vi "PH_PILS.ProcCases.vi"(0 "i ref in":refnum<vi>, 1 "selector":string, 2 "Data":T1, 3 "call cluster":T2={"Object"="", "Selector"="", "CallType"=enum."synchronous", "Async Object"="", "Async Selector"="", "Data Descriptor"="", "Data"=[], "Error #"=0, "Expire"=0}, 5 "error in (no error)":errorcluster) -> (14 "i ref out":refnum<vi>, 17 "answer cluster":T2={"Object"="", "Selector"="", "CallType"=enum."synchronous", "Async Object"="", "Async Selector"="", "Data Descriptor"="", "Data"=[], "Error #"=0, "Expire"=0}, 19 "error out":errorcluster)   [LabVIEW 2014, in "PH_PILS.lvlib"]
doc: "This method is called by a process from within the default case in the event loop. The methods of a class that are linked to events will be called from THIS method. Add your code here."
uses:
  PH_PILS.lvlib
  CSCore/CSSystem/CoreDefs/CoreDefs.call_type.ctl
  CSCore/BaseProcess/BaseProcess.descriptor string definition.ctl
  CSCore/CSSystem/CoreDefs/CoreDefs.rawDataType.ctl
  PH_SystemInformation/PH_SystemInformationEnabling State.ctl
  PH_Beckhoff_PP_Control/PH_Beckhoff_PP_Control.PP Mercury Tags.ctl
  CSCore/CSSystem/CoreLib/CoreLib.string 2 byte array.vi
  CSCore/BaseProcess/BaseProcess.lvlib
  CSCore/CSSystem/CoreLib/CoreLib.lvlib
  CSCore/CAEObj/CAEObj.lvlib
  PH_Common/PH_Common.lvlib
  PH_SystemInformation/PH_SystemInformation.lvlib
  PH_StatusHandler/PH_StatusHandler.lvlib
  PH_Beckhoff_PP_Control/PH_Beckhoff_PP_Control.lvlib
  PH_Beckhoff/PH_Beckhoff.lvlib
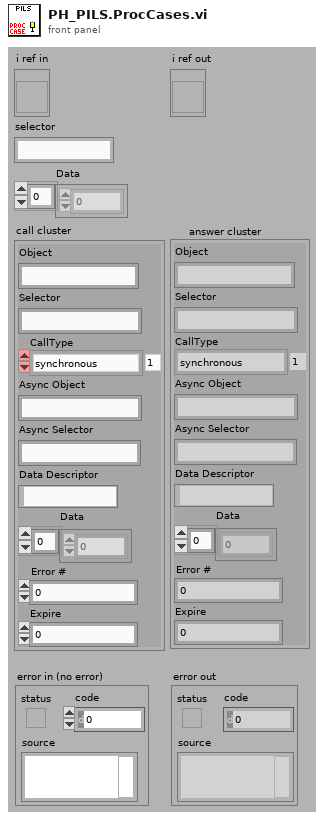
[diagram p1: front panel]
types:
  T1 = typedef "CoreDefs.rawDataType.ctl" = i8[]
  T2 = typedef "CoreDefs.call_type.ctl" = cluster{"Object":string, "Selector":string, "CallType":enum16{"simple", "synchronous", "asynchronous"}, "Async Object":string, "Async Selector":string, "Data Descriptor":T3, "Data":T1, "Error #":i32, "Expire":u32}
  T3 = typedef "BaseProcess.lvlib/BaseProcess.descriptor string definition.ctl" = string
  T4 = enum16{"unknown", "intern", "4 (Z6)", "3", "2", "1"}
  T5 = typedef "PH_Beckhoff_PP_Control.lvlib/PH_Beckhoff_PP_Control.PP Mercury Tags.ctl" = enum16{"Device-on", "Alarm", "on-since", "Concentration", "Status"}
  T6 = enum16{"Laser", "PreAmp", "MainAmp", "Exp 1", "Exp 2", "Exp 3", "Exp 4"}[]
  T7 = typedef "PH_SystemInformation.lvlib/PH_SystemInformationEnabling State.ctl" = i32
  T8 = typedef "PH_PILS.lvlib/PH_PILS.i attribute.ctl" = cluster{"Boolean":cluster{"GUI Ref":refnum<vi>, "Status":i32}[], "GUI Refs Exp. Shutters":cluster{"1":refnum<vi>, "2":refnum<vi>, "3":refnum<vi>, "4":refnum<vi>}, "Tristate2Run GUI Refs":refnum<vi>[], "EO-Likes":cluster{"GUI Ref":refnum<vi>, "Status":i32}[], "Operation Mode":cluster{"Operation Mode":T9, "GUI":cluster{"Ref State":refnum<vi>, "Ref":refnum<vi>}, "Servicemode":cluster{"Tagname":string, "Status":i32}, "Labormode":cluster{"Tagname":string, "Status":i32}, "Searchmode":cluster{"Tagname":string, "Status":i32}, "Shotmode":cluster{"Tagname":string, "Status":i32}}, "Submode":cluster{"Submode":T10, "GUI":cluster{"Ref State":refnum<vi>, "Ref":refnum<vi>}, "Submode":cluster{"Tagname":string, "Status":i32}}, "Experiment":cluster{"Experiment":enum16{"unknown", "intern", "4 (Z6)", "3", "2", "1"}, "GUI":cluster{"Ref State":refnum<vi>, "Ref":refnum<vi>}, "intern":cluster{"Tagname":string, "Status":i32}, "Exp 4":cluster{"Tagname":string, "Status":i32}, "Exp 3":cluster{"Tagname":string, "Status":i32}, "Exp 2":cluster{"Tagname":string, "Status":i32}, "Exp 1":cluster{"Tagname":string, "Status":i32}}, "TristateNormal":cluster{"GUI Ref":refnum<vi>, "Status":i32}[], "Door Tags":cluster{"GUI Ref":refnum<vi>, "Status":i32}[], "GUIlessTags":cluster{"Name":string, "Status":i32}[], "Beamline GUI Refs":refnum<vi>[], "Special Boolean":cluster{"GUI Ref":refnum<vi>, "Status":i32}[], "Laserpower":cluster{"GUI Ref":refnum<vi>, "Status":i32}[], "Shutter":cluster{"GUI Ref":refnum<vi>, "Status":i32}[], "Tristate EO Like":cluster{"GUI Ref":refnum<vi>, "Status":i32}[], "PP":cluster{"GUI Ref":refnum<vi>, "Status":i32, "Head Ref":refnum<vi>, "Slider Ref":refnum<vi>}[], "Switch Knobs":cluster{"GUI Ref":refnum<vi>, "Status":i32}[], "Latch Knob GUI Refs":refnum<vi>[], "FailureCounter":i32, "Enabled Status":cluster{"Laser":i32, "PreAmp":i32, "MainAmp":i32}, "Mercury":refnum<vi>, "Instance Rods":string, "Logfile":path, "Beckhoff-Instance Internal":string, "Beckhoff-Instance External":string, "Enabling Rights":cluster{"Name":string, "Password":string, "PA?":bool, "MA?":bool, "Exp?":bool}[]}
  T9 = typedef "PH_PILS.lvlib/PH_PILS.Operation Mode.ctl" = enum16{"unknown", "Service", "Labor", "Search", "Shot"}
  T10 = typedef "PH_PILS.lvlib/PH_PILS.Submode.ctl" = enum16{"unknown", "HV-Normal", "HV-Test"}
  T11 = enum16{"unknown", "intern", "4 (Z6)", "3", "2", "1"}[]
  T12 = typedef "PH_StatusHandler.lvlib/PH_StatusHandler.Status.ctl" = i16
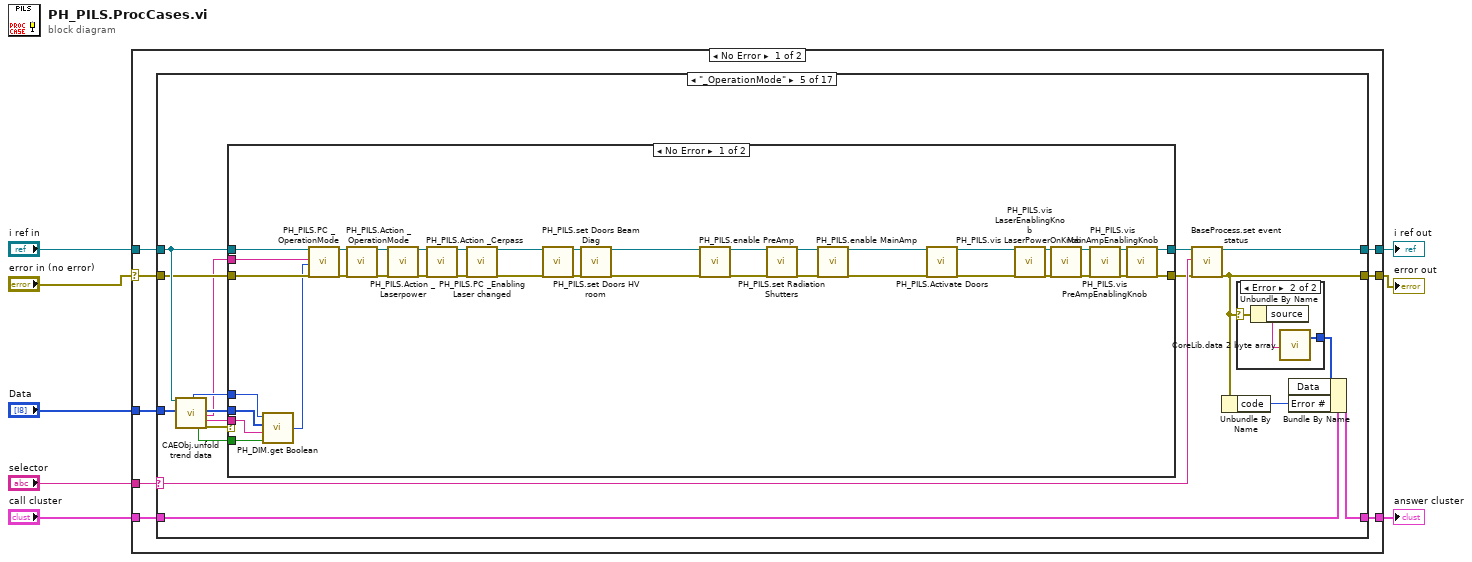
[diagram p0: block diagram]
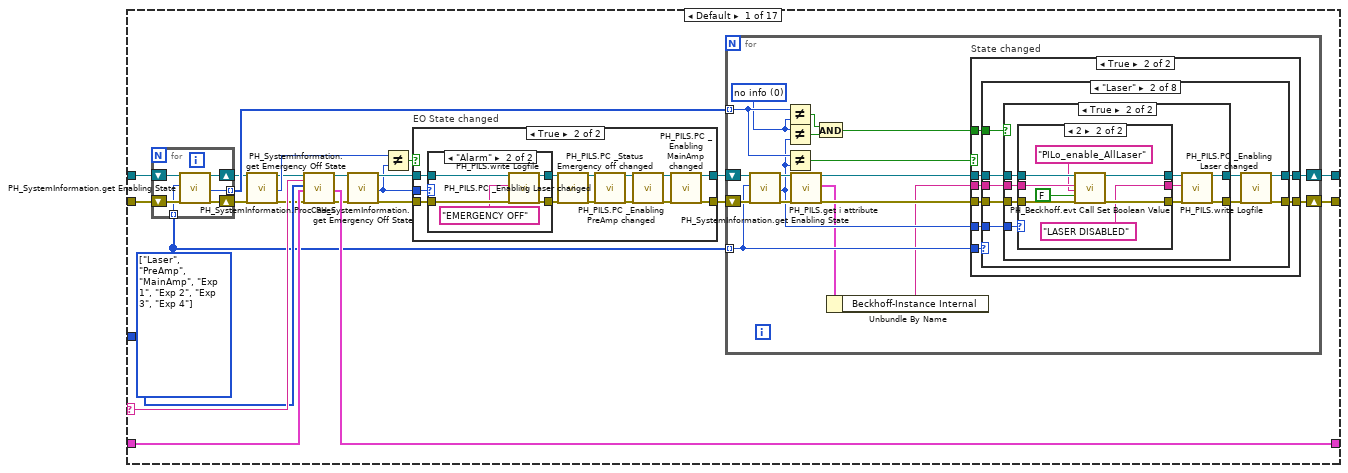
[diagram p2: hidden frame]
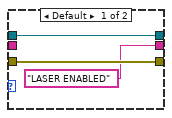
[diagram p6: hidden frame]
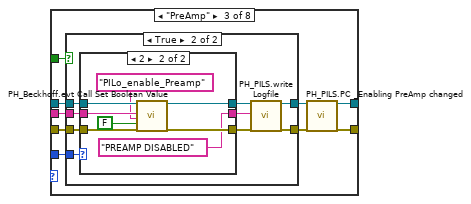
[diagram p7: hidden frame]
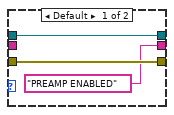
[diagram p9: hidden frame]
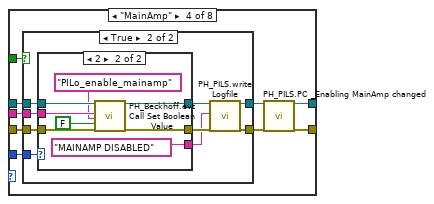
[diagram p10: hidden frame]
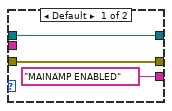
[diagram p12: hidden frame]
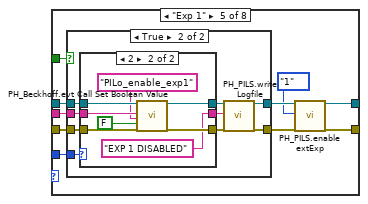
[diagram p13: hidden frame]
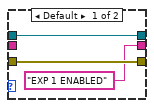
[diagram p15: hidden frame]
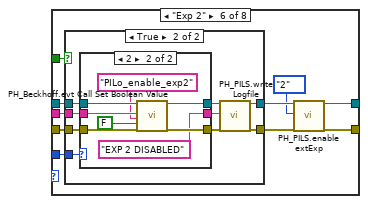
[diagram p16: hidden frame]
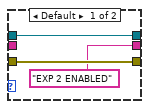
[diagram p18: hidden frame]
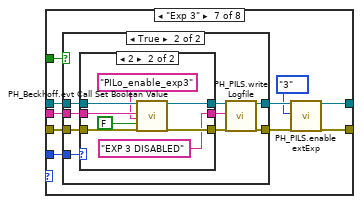
[diagram p19: hidden frame]
diagram:
  n1 = case shown="No Error" "error in (no error)" {
    selector: "error in (no error)" -> [w9 w1041]
    tunnel: "selector" -> [w16 _]
    tunnel: [w15 w1040] -> w7
    tunnel: "call cluster" -> [w14 w1040]
    tunnel: "i ref in" -> [w13 w1042]
    tunnel: [w12 w1042] -> w4
    tunnel: [w11 w1041] -> w3
    tunnel: "Data" -> [w10 _]
    frame No Error {
      n2 = case shown="\"_OperationMode\"" w16 {
        selector: w16 -> [w37 w334 w381 w416 w455 w516 w557 w606 w641 w676 w732 w779 w818 w851 w914 w955 w988]
        tunnel: w13 -> [w25 w328 w375 w410 w449 w510 w551 w600 w635 w670 w726 w773 w812 w845 w908 w949 w982]
        tunnel: [w34 w332 w379 w414 w453 w514 w555 w604 w639 w674 w730 w777 w816 w849 w912 w953 w986] -> w12
        tunnel: w14 -> [w38 w330 w377 w412 w451 w512 w553 w602 w637 w672 w728 w775 w814 w847 w910 w951 w984]
        tunnel: [w39 w329 w376 w411 w450 w511 w552 w601 w636 w671 w727 w774 w813 w846 w909 w950 w983] -> w15
        tunnel: w9 -> [w24 w327 w374 w409 w448 w509 w550 w599 w634 w669 w725 w772 w811 w844 w907 w948 w981]
        tunnel: [w33 w331 w378 w413 w452 w513 w554 w603 w638 w673 w729 w776 w815 w848 w911 w952 w985] -> w11
        tunnel: w10 -> [w31 w333 w380 w415 w454 w515 w556 w605 w640 w675 w731 w778 w817 w850 w913 w954 w987]
        frame Default {
          w17 = T6 [enum."Laser", enum."PreAmp", enum."MainAmp", enum."Exp 1", enum."Exp 2", enum."Exp 3", enum."Exp 4"] items=["Laser", "PreAmp", "MainAmp", "Exp 1", "Exp 2", "Exp 3", "Exp 4"]
          n3 = for {
            tunnel: [w314] -> w32 mode=indexing
            shift-right: [w317] -> w20
            shift-left: w25 -> [w318]
            shift-right: [w315] -> w22
            shift-left: w24 -> [w316]
            tunnel: w17 -> [w313] mode=indexing
            n4 = call "PH_SystemInformation.get Enabling State.vi"("i ref in"=w318, "Wanted State"=w313, "error in (no error)"=w316) -> ("i ref out"=w317:refnum<vi>, "Enabling State"=w314:T7, "error out"=w315:errorcluster)  [unwired: 14 in]
          }
          n5 = call "PH_SystemInformation.get Emergency Off State.vi"("i ref in"=w20, "error in (no error)"=w22) -> ("i ref out"=w19:refnum<vi>, "Emergency Off State"=w23:enum16{"no info", "off/false", "Alarm"}, "error out"=w21:errorcluster)  [unwired: 15 in]
          n6 = call "PH_SystemInformation.ProcCases.vi"("i ref in"=w19, "selector"=w37, "Data"=w31, "call cluster"=w38, "error in (no error)"=w21) -> ("i ref out"=w35:refnum<vi>, "answer cluster"=w39:T2, "error out"=w36:errorcluster)  [unwired: 12 in]
          n7 = call "PH_SystemInformation.get Emergency Off State.vi"("i ref in"=w35, "error in (no error)"=w36) -> ("i ref out"=w30:refnum<vi>, "Emergency Off State"=w18:enum16{"no info", "off/false", "Alarm"}, "error out"=w28:errorcluster)  [unwired: 15 in]
          n8 = Not Equal?(x=w23, y=w18) -> (x != y?=w26:bool)
          n9 = case "EO State changed" shown="True" w26 {
            tunnel: w30 -> [w292 w304]
            tunnel: [w292 w294] -> w29
            tunnel: w28 -> [w291 w305]
            tunnel: [w291 w293] -> w27
            tunnel: w18 -> [_ w303]
            frame False {
            }
            frame True {
              n10 = case shown="\"Alarm\"" w303 {
                tunnel: w305 -> [w306 w312]
                tunnel: [w306 w311] -> w301
                tunnel: w304 -> [w307 w310]
                tunnel: [w307 w309] -> w302
                frame Default {
                }
                frame "Alarm" {
                  n11 = call "PH_PILS.write Logfile.vi"("i ref in"=w310, "Text"="EMERGENCY OFF" ("string"), "error in"=w312) -> ("i ref out"=w309:refnum<vi>, "error out"=w311:errorcluster)  [unwired: 15 in]
                }
              }
              n12 = call "PH_PILS.PC _Status Emergency off changed.vi"("i ref in"=w302, "error in"=w301) -> ("i ref out"=w300:refnum<vi>, "error out"=w299:errorcluster)  [unwired: 16 in]
              n13 = call "PH_PILS.PC _Enabling Laser changed.vi"("i ref in"=w300, "error in"=w299) -> ("i ref out"=w298:refnum<vi>, "error out"=w297:errorcluster)  [unwired: 16 in]
              n14 = call "PH_PILS.PC _Enabling PreAmp changed.vi"("i ref in"=w298, "error in"=w297) -> ("i ref out"=w296:refnum<vi>, "error out"=w295:errorcluster)  [unwired: 16 in]
              n15 = call "PH_PILS.PC _Enabling MainAmp changed.vi"("i ref in"=w296, "error in"=w295) -> ("i ref out"=w294:refnum<vi>, "error out"=w293:errorcluster)  [unwired: 16 in]
            }
          }
          n16 = for {
            tunnel: w32 -> [w47] mode=indexing
            tunnel: w17 -> [w52] mode=indexing
            shift-right: [w54] -> w34
            shift-left: w29 -> [w57]
            shift-right: [w55] -> w33
            shift-left: w27 -> [w56]
            w43 = T7 0 items=["no info", "not disabled", "disabled"] ("Enabling State")
            n17 = call "PH_SystemInformation.get Enabling State.vi"("i ref in"=w57, "Wanted State"=w52, "error in (no error)"=w56) -> ("i ref out"=w50:refnum<vi>, "Enabling State"=w46:T7, "error out"=w51:errorcluster)  [unwired: 14 in]
            n18 = Not Equal?(x=w47, y=w43) -> (x != y?=w45:bool)
            n19 = Not Equal?(x=w43, y=w46) -> (x != y?=w44:bool)
            n20 = Not Equal?(x=w47, y=w46) -> (x != y?=w53:bool)
            n21 = call "PH_PILS.get i attribute.vi"("i ref in"=w50, "error in (no error)"=w51) -> ("i ref out"=w49:refnum<vi>, "i attribute"=w40:T8, "error out"=w48:errorcluster)  [unwired: 15 in]
            n22 = And(x=w45, y=w44) -> (x .and. y?=w42:bool)
            n23 = Unbundle By Name(w40) -> ("Beckhoff-Instance Internal"=w41:string)
            n24 = case "State changed" shown="True" w53 {
              tunnel: w48 -> [w58 w67]
              tunnel: [w58 w66] -> w55
              tunnel: w49 -> [w59 w65]
              tunnel: [w59 w64] -> w54
              tunnel: w52 -> [_ w63]
              tunnel: w46 -> [_ w62]
              tunnel: w41 -> [_ w61]
              tunnel: w42 -> [_ w60]
              frame False {
              }
              frame True {
                n25 = case shown="\"Laser\"" w63 {
                  tunnel: w67 -> [w68 w75 w108 w139 w171 w203 w235 w267]
                  tunnel: [w68 w78 w101 w132 w164 w196 w228 w260] -> w66
                  tunnel: w65 -> [w69 w76 w109 w140 w172 w204 w236 w268]
                  tunnel: [w69 w77 w102 w133 w166 w198 w230 w262] -> w64
                  tunnel: w62 -> [_ w73 w106 w137 w169 w201 w233 w265]
                  tunnel: w61 -> [_ w74 w107 w138 w170 w202 w234 w266]
                  tunnel: w60 -> [_ w72 w105 w136 w168 w200 w232 w264]
                  frame Default {
                  }
                  frame "Laser" {
                    n26 = case shown="True" w72 {
                      tunnel: w76 -> [w80 w89]
                      tunnel: [w80 w84] -> w71
                      tunnel: w75 -> [w79 w88]
                      tunnel: [w79 w82] -> w70
                      tunnel: w74 -> [_ w87]
                      tunnel: w73 -> [_ w86]
                      frame False {
                      }
                      frame True {
                        n27 = case shown="2" w86 {
                          tunnel: w89 -> [w92 w100]
                          tunnel: [w92 w99] -> w85
                          tunnel: w88 -> [w91 w98]
                          tunnel: [w91 w97] -> w83
                          tunnel: w87 -> [_ w96]
                          tunnel: ["LASER ENABLED" ("string") "LASER DISABLED" ("string")] -> w81
                          frame Default {
                          }
                          frame 2 {
                            n28 = call "PH_Beckhoff.evt Call Set Boolean Value.vi"("i ref in"=w100, "Beckhoff Instance"=w96, "Tagname to set"="PILo_enable_AllLaser", "Value"=FALSE ("Value to set"), "error in"=w98) -> ("i ref out"=w99:refnum<vi>, "error out"=w97:errorcluster)  [unwired: 13 in]
                          }
                        }
                        n29 = call "PH_PILS.write Logfile.vi"("i ref in"=w85, "Text"=w81, "error in"=w83) -> ("i ref out"=w84:refnum<vi>, "error out"=w82:errorcluster)  [unwired: 15 in]
                      }
                    }
                    n30 = call "PH_PILS.PC _Enabling Laser changed.vi"("i ref in"=w71, "error in"=w70) -> ("i ref out"=w77:refnum<vi>, "error out"=w78:errorcluster)  [unwired: 16 in]
                  }
                  frame "PreAmp" {
                    n31 = case shown="True" w105 {
                      tunnel: w109 -> [w111 w120]
                      tunnel: w108 -> [w110 w119]
                      tunnel: w107 -> [_ w118]
                      tunnel: w106 -> [_ w117]
                      tunnel: [w111 w115] -> w104
                      tunnel: [w110 w113] -> w103
                      frame False {
                      }
                      frame True {
                        n32 = case shown="2" w117 {
                          tunnel: w120 -> [w123 w131]
                          tunnel: [w123 w130] -> w116
                          tunnel: w119 -> [w122 w129]
                          tunnel: [w122 w128] -> w114
                          tunnel: w118 -> [_ w127]
                          tunnel: ["PREAMP ENABLED" ("string") "PREAMP DISABLED" ("string")] -> w112
                          frame Default {
                          }
                          frame 2 {
                            n33 = call "PH_Beckhoff.evt Call Set Boolean Value.vi"("i ref in"=w131, "Beckhoff Instance"=w127, "Tagname to set"="PILo_enable_Preamp", "Value"=FALSE ("Value to set"), "error in"=w129) -> ("i ref out"=w130:refnum<vi>, "error out"=w128:errorcluster)  [unwired: 13 in]
                          }
                        }
                        n34 = call "PH_PILS.write Logfile.vi"("i ref in"=w116, "Text"=w112, "error in"=w114) -> ("i ref out"=w115:refnum<vi>, "error out"=w113:errorcluster)  [unwired: 15 in]
                      }
                    }
                    n35 = call "PH_PILS.PC _Enabling PreAmp changed.vi"("i ref in"=w104, "error in"=w103) -> ("i ref out"=w102:refnum<vi>, "error out"=w101:errorcluster)  [unwired: 16 in]
                  }
                  frame "MainAmp" {
                    n36 = case shown="True" w136 {
                      tunnel: w140 -> [w142 w151]
                      tunnel: w139 -> [w141 w150]
                      tunnel: w138 -> [_ w149]
                      tunnel: w137 -> [_ w148]
                      tunnel: [w142 w146] -> w135
                      tunnel: [w141 w144] -> w134
                      frame False {
                      }
                      frame True {
                        n37 = case shown="2" w148 {
                          tunnel: w151 -> [w154 w162]
                          tunnel: [w154 w161] -> w147
                          tunnel: w150 -> [w153 w160]
                          tunnel: [w153 w159] -> w145
                          tunnel: w149 -> [_ w158]
                          tunnel: ["MAINAMP ENABLED" ("string") "MAINAMP DISABLED" ("string")] -> w143
                          frame Default {
                          }
                          frame 2 {
                            n38 = call "PH_Beckhoff.evt Call Set Boolean Value.vi"("i ref in"=w162, "Beckhoff Instance"=w158, "Tagname to set"="PILo_enable_mainamp", "Value"=FALSE ("Value to set"), "error in"=w160) -> ("i ref out"=w161:refnum<vi>, "error out"=w159:errorcluster)  [unwired: 13 in]
                          }
                        }
                        n39 = call "PH_PILS.write Logfile.vi"("i ref in"=w147, "Text"=w143, "error in"=w145) -> ("i ref out"=w146:refnum<vi>, "error out"=w144:errorcluster)  [unwired: 15 in]
                      }
                    }
                    n40 = call "PH_PILS.PC _Enabling MainAmp changed.vi"("i ref in"=w135, "error in"=w134) -> ("i ref out"=w133:refnum<vi>, "error out"=w132:errorcluster)  [unwired: 16 in]
                  }
                  frame "Exp 1" {
                    n41 = case shown="True" w168 {
                      tunnel: w172 -> [w174 w183]
                      tunnel: w171 -> [w173 w182]
                      tunnel: w170 -> [_ w181]
                      tunnel: w169 -> [_ w180]
                      tunnel: [w174 w178] -> w167
                      tunnel: [w173 w176] -> w165
                      frame False {
                      }
                      frame True {
                        n42 = case shown="2" w180 {
                          tunnel: w183 -> [w186 w194]
                          tunnel: [w186 w193] -> w179
                          tunnel: w182 -> [w185 w192]
                          tunnel: [w185 w191] -> w177
                          tunnel: w181 -> [_ w190]
                          tunnel: ["EXP 1 ENABLED" ("string") "EXP 1 DISABLED" ("string")] -> w175
                          frame Default {
                          }
                          frame 2 {
                            n43 = call "PH_Beckhoff.evt Call Set Boolean Value.vi"("i ref in"=w194, "Beckhoff Instance"=w190, "Tagname to set"="PILo_enable_exp1", "Value"=FALSE ("Value to set"), "error in"=w192) -> ("i ref out"=w193:refnum<vi>, "error out"=w191:errorcluster)  [unwired: 13 in]
                          }
                        }
                        n44 = call "PH_PILS.write Logfile.vi"("i ref in"=w179, "Text"=w175, "error in"=w177) -> ("i ref out"=w178:refnum<vi>, "error out"=w176:errorcluster)  [unwired: 15 in]
                      }
                    }
                    n45 = call "PH_PILS.enable extExp.vi"("i ref in"=w167, "Experiment.Experiment"=T4."1", "error in"=w165) -> ("i ref out"=w166:refnum<vi>, "error out"=w164:errorcluster)  [unwired: 15 in]
                  }
                  frame "Exp 2" {
                    n46 = case shown="True" w200 {
                      tunnel: w204 -> [w206 w215]
                      tunnel: w203 -> [w205 w214]
                      tunnel: w202 -> [_ w213]
                      tunnel: w201 -> [_ w212]
                      tunnel: [w206 w210] -> w199
                      tunnel: [w205 w208] -> w197
                      frame False {
                      }
                      frame True {
                        n47 = case shown="2" w212 {
                          tunnel: w215 -> [w218 w226]
                          tunnel: [w218 w225] -> w211
                          tunnel: w214 -> [w217 w224]
                          tunnel: [w217 w223] -> w209
                          tunnel: w213 -> [_ w222]
                          tunnel: ["EXP 2 ENABLED" ("string") "EXP 2 DISABLED" ("string")] -> w207
                          frame Default {
                          }
                          frame 2 {
                            n48 = call "PH_Beckhoff.evt Call Set Boolean Value.vi"("i ref in"=w226, "Beckhoff Instance"=w222, "Tagname to set"="PILo_enable_exp2", "Value"=FALSE ("Value to set"), "error in"=w224) -> ("i ref out"=w225:refnum<vi>, "error out"=w223:errorcluster)  [unwired: 13 in]
                          }
                        }
                        n49 = call "PH_PILS.write Logfile.vi"("i ref in"=w211, "Text"=w207, "error in"=w209) -> ("i ref out"=w210:refnum<vi>, "error out"=w208:errorcluster)  [unwired: 15 in]
                      }
                    }
                    n50 = call "PH_PILS.enable extExp.vi"("i ref in"=w199, "Experiment.Experiment"=T4."2", "error in"=w197) -> ("i ref out"=w198:refnum<vi>, "error out"=w196:errorcluster)  [unwired: 15 in]
                  }
                  frame "Exp 3" {
                    n51 = case shown="True" w232 {
                      tunnel: w236 -> [w238 w247]
                      tunnel: w235 -> [w237 w246]
                      tunnel: w234 -> [_ w245]
                      tunnel: w233 -> [_ w244]
                      tunnel: [w238 w240] -> w231
                      tunnel: [w237 w242] -> w229
                      frame False {
                      }
                      frame True {
                        n52 = case shown="2" w244 {
                          tunnel: w247 -> [w250 w258]
                          tunnel: [w250 w253] -> w241
                          tunnel: w246 -> [w249 w257]
                          tunnel: [w249 w252] -> w243
                          tunnel: w245 -> [_ w256]
                          tunnel: ["EXP 3 ENABLED" ("string") "EXP 3 DISABLED" ("string")] -> w239
                          frame Default {
                          }
                          frame 2 {
                            n53 = call "PH_Beckhoff.evt Call Set Boolean Value.vi"("i ref in"=w258, "Beckhoff Instance"=w256, "Tagname to set"="PILo_enable_exp3", "Value"=FALSE ("Value to set"), "error in"=w257) -> ("i ref out"=w253:refnum<vi>, "error out"=w252:errorcluster)  [unwired: 13 in]
                          }
                        }
                        n54 = call "PH_PILS.write Logfile.vi"("i ref in"=w241, "Text"=w239, "error in"=w243) -> ("i ref out"=w240:refnum<vi>, "error out"=w242:errorcluster)  [unwired: 15 in]
                      }
                    }
                    n55 = call "PH_PILS.enable extExp.vi"("i ref in"=w231, "Experiment.Experiment"=T4."3", "error in"=w229) -> ("i ref out"=w230:refnum<vi>, "error out"=w228:errorcluster)  [unwired: 15 in]
                  }
                  frame "Exp 4" {
                    n56 = case shown="True" w264 {
                      tunnel: w268 -> [w270 w279]
                      tunnel: w267 -> [w269 w278]
                      tunnel: w266 -> [_ w277]
                      tunnel: w265 -> [_ w276]
                      tunnel: [w270 w274] -> w263
                      tunnel: [w269 w272] -> w261
                      frame False {
                      }
                      frame True {
                        n57 = case shown="2" w276 {
                          tunnel: w279 -> [w282 w290]
                          tunnel: [w282 w289] -> w275
                          tunnel: w278 -> [w281 w288]
                          tunnel: [w281 w287] -> w273
                          tunnel: w277 -> [_ w286]
                          tunnel: ["EXP 4 (Z6) ENABLED" ("string") "EXP 4 (Z6) DISABLED" ("string")] -> w271
                          frame Default {
                          }
                          frame 2 {
                            n58 = call "PH_Beckhoff.evt Call Set Boolean Value.vi"("i ref in"=w290, "Beckhoff Instance"=w286, "Tagname to set"="PILo_enable_exp4", "Value"=FALSE ("Value to set"), "error in"=w288) -> ("i ref out"=w289:refnum<vi>, "error out"=w287:errorcluster)  [unwired: 13 in]
                          }
                        }
                        n59 = call "PH_PILS.write Logfile.vi"("i ref in"=w275, "Text"=w271, "error in"=w273) -> ("i ref out"=w274:refnum<vi>, "error out"=w272:errorcluster)  [unwired: 15 in]
                      }
                    }
                    n60 = call "PH_PILS.enable extExp.vi"("i ref in"=w263, "Experiment.Experiment"=T4."4 (Z6)", "error in"=w261) -> ("i ref out"=w262:refnum<vi>, "error out"=w260:errorcluster)  [unwired: 15 in]
                  }
                }
              }
            }
          }
        }
        frame "_EO_Likes" {
          n61 = call "CAEObj.unfold trend data.vi"("i ref in"=w328, "raw trend data"=w333) -> ("quality"=w321:i32, "no link"=w323:bool, "data"=w322:i8[], "serviceName"=w319:string, "typeDescriptor"=w320:string, "error out"=w324:errorcluster)  [unwired: 9 in, 3 out]
          n62 = case shown="No Error" w324 {
            tunnel: w327 -> [w360 w361]
            tunnel: [w343 w362] -> w325
            tunnel: [w341 w361] -> w326
            tunnel: w328 -> [w359 w362]
            tunnel: w323 -> [w356 _]
            tunnel: w320 -> [w354 _]
            tunnel: w322 -> [w358 _]
            tunnel: w321 -> [w357 _]
            tunnel: w319 -> [w353 _]
            frame No Error {
              n63 = call "PH_DIM.get Boolean.vi"("no link"=w356, "typeDescriptor"=w354, "data"=w358, "quality"=w357) -> ("Value"=w355:i32)
              n64 = call "PH_PILS.PC _EOLikes.vi"("i ref in"=w359, "serviceName"=w353, "Value"=w355, "error IO"=w360) -> ("i ref out"=w352:refnum<vi>, "error out"=w351:errorcluster)  [unwired: 14 in]
              n65 = call "PH_PILS.enable PreAmp.vi"("i ref in"=w352, "error in"=w351) -> ("i ref out"=w350:refnum<vi>, "error out"=w349:errorcluster)  [unwired: 16 in]
              n66 = call "PH_PILS.enable MainAmp.vi"("i ref in"=w350, "error in"=w349) -> ("i ref out"=w340:refnum<vi>, "error out"=w338:errorcluster)  [unwired: 16 in]
              n67 = call "PH_PILS.set Radiation Shutters.vi"("i ref in"=w340, "error in"=w338) -> ("i ref out"=w339:refnum<vi>, "error out"=w337:errorcluster)  [unwired: 16 in]
              n68 = call "PH_PILS.vis HVroomLockKnob.vi"("i ref in"=w339, "error IO"=w337) -> ("i ref out"=w348:refnum<vi>, "error out"=w347:errorcluster)  [unwired: 16 in]
              n69 = call "PH_PILS.vis PreAmpEnablingKnob.vi"("i ref in"=w348, "error IO"=w347) -> ("i ref out"=w345:refnum<vi>, "error out"=w346:errorcluster)  [unwired: 16 in]
              n70 = call "PH_PILS.vis MainAmpEnablingKnob.vi"("i ref in"=w345, "error IO"=w346) -> ("i ref out"=w344:refnum<vi>, "error out"=w342:errorcluster)  [unwired: 16 in]
              n71 = call "PH_PILS.vis ResetExtEOKnob.vi"("i ref in"=w344, "error IO"=w342) -> ("i ref out"=w343:refnum<vi>, "error out"=w341:errorcluster)  [unwired: 16 in]
            }
            frame Error {
            }
          }
          n72 = call "BaseProcess.set event status.vi"("i ref in"=w325, "EventStatus"=w334, "error in (no error)"=w326) -> ("i ref out"=w332:refnum<vi>, "error out"=w331:errorcluster)  [unwired: 14 in, 1 out]
          n73 = Unbundle By Name(w331) -> ("code"=w335:i32)
          n74 = case shown="Error" w331 {
            selector: w331 -> [_ w365]
            tunnel: [_ w363] -> w336
            frame No Error {
            }
            frame Error {
              n75 = Unbundle By Name(w365) -> ("source"=w364:string)
              n76 = call-poly "CoreLib.data 2 byte array.vi"("string"=w364) -> ("byteArray out"=w363:T1)  [unwired: 18 in]
            }
          }
          n77 = Bundle By Name(cluster=w330, "Data"=w336, "Error #"=w335) -> (w329:T2)
        }
        frame "_Laserpower" {
          n78 = call "CAEObj.unfold trend data.vi"("i ref in"=w375, "raw trend data"=w380) -> ("quality"=w368:i32, "no link"=w370:bool, "data"=w369:i8[], "serviceName"=w366:string, "typeDescriptor"=w367:string, "error out"=w371:errorcluster)  [unwired: 9 in, 3 out]
          n79 = case shown="No Error" w371 {
            tunnel: w374 -> [w390 w396]
            tunnel: [w384 w397] -> w372
            tunnel: [w386 w396] -> w373
            tunnel: w375 -> [w391 w397]
            tunnel: w370 -> [w393 _]
            tunnel: w367 -> [w392 _]
            tunnel: w369 -> [w395 _]
            tunnel: w368 -> [w394 _]
            tunnel: w366 -> [w388 _]
            frame No Error {
              n80 = call "PH_DIM.get Boolean.vi"("no link"=w393, "typeDescriptor"=w392, "data"=w395, "quality"=w394) -> ("Value"=w387:i32)
              n81 = call "PH_PILS.PC _Laserpower.vi"("i ref in"=w391, "serviceName"=w388, "Value"=w387, "error IO"=w390) -> ("i ref out"=w385:refnum<vi>, "error out"=w389:errorcluster)  [unwired: 14 in]
              n82 = call "PH_PILS.Action _Laserpower.vi"("i ref in"=w385, "error in"=w389) -> ("i ref out"=w384:refnum<vi>, "error out"=w386:errorcluster)  [unwired: 16 in]
            }
            frame Error {
            }
          }
          n83 = call "BaseProcess.set event status.vi"("i ref in"=w372, "EventStatus"=w381, "error in (no error)"=w373) -> ("i ref out"=w379:refnum<vi>, "error out"=w378:errorcluster)  [unwired: 14 in, 1 out]
          n84 = case shown="No Error" w378 {
            selector: w378 -> [_ w400]
            tunnel: [_ w398] -> w383
            frame No Error {
            }
            frame Error {
              n85 = Unbundle By Name(w400) -> ("source"=w399:string)
              n86 = call-poly "CoreLib.data 2 byte array.vi"("string"=w399) -> ("byteArray out"=w398:T1)  [unwired: 18 in]
            }
          }
          n87 = Unbundle By Name(w378) -> ("code"=w382:i32)
          n88 = Bundle By Name(cluster=w377, "Data"=w383, "Error #"=w382) -> (w376:T2)
        }
        frame "_GUILessTags" {
          n89 = call "CAEObj.unfold trend data.vi"("i ref in"=w410, "raw trend data"=w415) -> ("quality"=w404:i32, "no link"=w406:bool, "data"=w405:i8[], "serviceName"=w402:string, "typeDescriptor"=w403:string, "error out"=w407:errorcluster)  [unwired: 9 in, 3 out]
          n90 = case shown="No Error" w407 {
            tunnel: w409 -> [w434 w435]
            tunnel: [w419 w436] -> w401
            tunnel: [w421 w435] -> w408
            tunnel: w410 -> [w433 w436]
            tunnel: w406 -> [w430 _]
            tunnel: w403 -> [w429 _]
            tunnel: w405 -> [w432 _]
            tunnel: w404 -> [w431 _]
            tunnel: w402 -> [w426 _]
            frame No Error {
              n91 = call "PH_DIM.get Boolean.vi"("no link"=w430, "typeDescriptor"=w429, "data"=w432, "quality"=w431) -> ("Value"=w427:i32)
              n92 = call "PH_PILS.PC _GUILessTags.vi"("i ref in"=w433, "serviceName"=w426, "Value"=w427, "error IO"=w434) -> ("i ref out"=w425:refnum<vi>, "error out"=w428:errorcluster)  [unwired: 14 in]
              n93 = call "PH_PILS.set color of beamline.vi"("i ref in"=w425, "error in"=w428) -> ("i ref out"=w424:refnum<vi>, "error out"=w423:errorcluster)  [unwired: 16 in]
              n94 = call "PH_PILS.vis LaserPowerOnKnob.vi"("i ref in"=w424, "error IO"=w423) -> ("i ref out"=w420:refnum<vi>, "error out"=w422:errorcluster)  [unwired: 16 in]
              n95 = call "PH_PILS.vis MainAmpEnablingKnob.vi"("i ref in"=w420, "error IO"=w422) -> ("i ref out"=w419:refnum<vi>, "error out"=w421:errorcluster)  [unwired: 16 in]
            }
            frame Error {
            }
          }
          n96 = call "BaseProcess.set event status.vi"("i ref in"=w401, "EventStatus"=w416, "error in (no error)"=w408) -> ("i ref out"=w414:refnum<vi>, "error out"=w413:errorcluster)  [unwired: 14 in, 1 out]
          n97 = case shown="No Error" w413 {
            selector: w413 -> [_ w439]
            tunnel: [_ w437] -> w418
            frame No Error {
            }
            frame Error {
              n98 = Unbundle By Name(w439) -> ("source"=w438:string)
              n99 = call-poly "CoreLib.data 2 byte array.vi"("string"=w438) -> ("byteArray out"=w437:T1)  [unwired: 18 in]
            }
          }
          n100 = Unbundle By Name(w413) -> ("code"=w417:i32)
          n101 = Bundle By Name(cluster=w412, "Data"=w418, "Error #"=w417) -> (w411:T2)
        }
        frame "_OperationMode" {
          n102 = call "CAEObj.unfold trend data.vi"("i ref in"=w449, "raw trend data"=w454) -> ("quality"=w442:i32, "no link"=w444:bool, "data"=w443:i8[], "serviceName"=w440:string, "typeDescriptor"=w441:string, "error out"=w445:errorcluster)  [unwired: 9 in, 3 out]
          n103 = case shown="No Error" w445 {
            tunnel: w448 -> [w495 w496]
            tunnel: [w474 w497] -> w446
            tunnel: [w476 w496] -> w447
            tunnel: w449 -> [w494 w497]
            tunnel: w444 -> [w491 _]
            tunnel: w441 -> [w490 _]
            tunnel: w443 -> [w493 _]
            tunnel: w442 -> [w492 _]
            tunnel: w440 -> [w488 _]
            frame No Error {
              n104 = call "PH_DIM.get Boolean.vi"("no link"=w491, "typeDescriptor"=w490, "data"=w493, "quality"=w492) -> ("Value"=w487:i32)
              n105 = call "PH_PILS.PC _OperationMode.vi"("i ref in"=w494, "Servicename"=w488, "Value"=w487, "error IO"=w495) -> ("i ref out"=w486:refnum<vi>, "error out"=w489:errorcluster)  [unwired: 14 in]
              n106 = call "PH_PILS.Action _OperationMode.vi"("i ref in"=w486, "error IO"=w489) -> ("i ref out"=w473:refnum<vi>, "error out"=w472:errorcluster)  [unwired: 16 in]
              n107 = call "PH_PILS.Action _Laserpower.vi"("i ref in"=w473, "error in"=w472) -> ("i ref out"=w485:refnum<vi>, "error out"=w484:errorcluster)  [unwired: 16 in]
              n108 = call "PH_PILS.Action _Cerpass.vi"("i ref in"=w485, "error in"=w484) -> ("i ref out"=w471:refnum<vi>, "error out"=w470:errorcluster)  [unwired: 16 in]
              n109 = call "PH_PILS.PC _Enabling Laser changed.vi"("i ref in"=w471, "error in"=w470) -> ("i ref out"=w469:refnum<vi>, "error out"=w468:errorcluster)  [unwired: 16 in]
              n110 = call "PH_PILS.set Doors Beam Diag.vi"("i ref in"=w469, "error in"=w468) -> ("i ref out"=w483:refnum<vi>, "error out"=w482:errorcluster)  [unwired: 16 in]
              n111 = call "PH_PILS.set Doors HV room.vi"("i ref in"=w483, "error in"=w482) -> ("i ref out"=w462:refnum<vi>, "error out"=w463:errorcluster)  [unwired: 16 in]
              n112 = call "PH_PILS.enable PreAmp.vi"("i ref in"=w462, "error in"=w463) -> ("i ref out"=w461:refnum<vi>, "error out"=w459:errorcluster)  [unwired: 16 in]
              n113 = call "PH_PILS.set Radiation Shutters.vi"("i ref in"=w461, "error in"=w459) -> ("i ref out"=w460:refnum<vi>, "error out"=w458:errorcluster)  [unwired: 16 in]
              n114 = call "PH_PILS.enable MainAmp.vi"("i ref in"=w460, "error in"=w458) -> ("i ref out"=w467:refnum<vi>, "error out"=w466:errorcluster)  [unwired: 16 in]
              n115 = call "PH_PILS.Activate Doors.vi"("i ref in"=w467, "error in (no error)"=w466) -> ("i ref out"=w465:refnum<vi>, "error out"=w464:errorcluster)  [unwired: 16 in]
              n116 = call "PH_PILS.vis LaserEnablingKnob.vi"("i ref in"=w465, "error IO"=w464) -> ("i ref out"=w481:refnum<vi>, "error out"=w480:errorcluster)  [unwired: 16 in]
              n117 = call "PH_PILS.vis LaserPowerOnKnob.vi"("i ref in"=w481, "error IO"=w480) -> ("i ref out"=w479:refnum<vi>, "error out"=w478:errorcluster)  [unwired: 16 in]
              n118 = call "PH_PILS.vis PreAmpEnablingKnob.vi"("i ref in"=w479, "error IO"=w478) -> ("i ref out"=w475:refnum<vi>, "error out"=w477:errorcluster)  [unwired: 16 in]
              n119 = call "PH_PILS.vis MainAmpEnablingKnob.vi"("i ref in"=w475, "error IO"=w477) -> ("i ref out"=w474:refnum<vi>, "error out"=w476:errorcluster)  [unwired: 16 in]
            }
            frame Error {
            }
          }
          n120 = call "BaseProcess.set event status.vi"("i ref in"=w446, "EventStatus"=w455, "error in (no error)"=w447) -> ("i ref out"=w453:refnum<vi>, "error out"=w452:errorcluster)  [unwired: 14 in, 1 out]
          n121 = Unbundle By Name(w452) -> ("code"=w456:i32)
          n122 = case shown="Error" w452 {
            selector: w452 -> [_ w500]
            tunnel: [_ w498] -> w457
            frame No Error {
            }
            frame Error {
              n123 = Unbundle By Name(w500) -> ("source"=w499:string)
              n124 = call-poly "CoreLib.data 2 byte array.vi"("string"=w499) -> ("byteArray out"=w498:T1)  [unwired: 18 in]
            }
          }
          n125 = Bundle By Name(cluster=w451, "Data"=w457, "Error #"=w456) -> (w450:T2)
        }
        frame "_Submode" {
          n126 = call "CAEObj.unfold trend data.vi"("i ref in"=w510, "raw trend data"=w515) -> ("quality"=w503:i32, "no link"=w505:bool, "data"=w504:i8[], "serviceName"=w501:string, "typeDescriptor"=w502:string, "error out"=w506:errorcluster)  [unwired: 9 in, 3 out]
          n127 = case shown="No Error" w506 {
            tunnel: w509 -> [w536 w537]
            tunnel: [w519 w538] -> w507
            tunnel: [w521 w537] -> w508
            tunnel: w510 -> [w535 w538]
            tunnel: w505 -> [w532 _]
            tunnel: w502 -> [w531 _]
            tunnel: w504 -> [w534 _]
            tunnel: w503 -> [w533 _]
            tunnel: w501 -> [w529 _]
            frame No Error {
              n128 = call "PH_DIM.get Boolean.vi"("no link"=w532, "typeDescriptor"=w531, "data"=w534, "quality"=w533) -> ("Value"=w528:i32)
              n129 = call "PH_PILS.PC _Subode.vi"("i ref in"=w535, "Servicename"=w529, "Value"=w528, "error IO"=w536) -> ("i ref out"=w527:refnum<vi>, "error out"=w530:errorcluster)  [unwired: 14 in]
              n130 = call "PH_PILS.Action _Submode.vi"("i ref in"=w527, "error IO"=w530) -> ("i ref out"=w526:refnum<vi>, "error out"=w525:errorcluster)  [unwired: 16 in]
              n131 = call "PH_PILS.set Doors HV room.vi"("i ref in"=w526, "error in"=w525) -> ("i ref out"=w524:refnum<vi>, "error out"=w523:errorcluster)  [unwired: 16 in]
              n132 = call "PH_PILS.enable MainAmp.vi"("i ref in"=w524, "error in"=w523) -> ("i ref out"=w520:refnum<vi>, "error out"=w522:errorcluster)  [unwired: 16 in]
              n133 = call "PH_PILS.vis MainAmpEnablingKnob.vi"("i ref in"=w520, "error IO"=w522) -> ("i ref out"=w519:refnum<vi>, "error out"=w521:errorcluster)  [unwired: 16 in]
            }
            frame Error {
            }
          }
          n134 = call "BaseProcess.set event status.vi"("i ref in"=w507, "EventStatus"=w516, "error in (no error)"=w508) -> ("i ref out"=w514:refnum<vi>, "error out"=w513:errorcluster)  [unwired: 14 in, 1 out]
          n135 = case shown="No Error" w513 {
            selector: w513 -> [_ w541]
            tunnel: [_ w539] -> w518
            frame No Error {
            }
            frame Error {
              n136 = Unbundle By Name(w541) -> ("source"=w540:string)
              n137 = call-poly "CoreLib.data 2 byte array.vi"("string"=w540) -> ("byteArray out"=w539:T1)  [unwired: 18 in]
            }
          }
          n138 = Unbundle By Name(w513) -> ("code"=w517:i32)
          n139 = Bundle By Name(cluster=w512, "Data"=w518, "Error #"=w517) -> (w511:T2)
        }
        frame "_Experiment" {
          n140 = call "CAEObj.unfold trend data.vi"("i ref in"=w551, "raw trend data"=w556) -> ("quality"=w544:i32, "no link"=w546:bool, "data"=w545:i8[], "serviceName"=w542:string, "typeDescriptor"=w543:string, "error out"=w547:errorcluster)  [unwired: 9 in, 3 out]
          n141 = case shown="No Error" w547 {
            tunnel: w550 -> [w580 w586]
            tunnel: [w561 w587] -> w548
            tunnel: [w563 w586] -> w549
            tunnel: w551 -> [w579 w587]
            tunnel: w546 -> [w576 _]
            tunnel: w543 -> [w575 _]
            tunnel: w545 -> [w578 _]
            tunnel: w544 -> [w577 _]
            tunnel: w542 -> [w573 _]
            frame No Error {
              w560 = T11 [enum."4 (Z6)", enum."3", enum."2", enum."1"] items=["unknown", "intern", "4 (Z6)", "3", "2", "1"]
              n142 = call "PH_DIM.get Boolean.vi"("no link"=w576, "typeDescriptor"=w575, "data"=w578, "quality"=w577) -> ("Value"=w572:i32)
              n143 = call "PH_PILS.PC _Experiment.vi"("i ref in"=w579, "Servicename"=w573, "Value"=w572, "error IO"=w580) -> ("i ref out"=w571:refnum<vi>, "error out"=w574:errorcluster)  [unwired: 14 in]
              n144 = call "PH_PILS.Action _Experiment.vi"("i ref in"=w571, "error IO"=w574) -> ("i ref out"=w570:refnum<vi>, "error out"=w569:errorcluster)  [unwired: 16 in]
              n145 = for {
                shift-right: [w583] -> w568
                shift-left: w570 -> [w585]
                shift-right: [w582] -> w567
                shift-left: w569 -> [w584]
                tunnel: w560 -> [w581] mode=indexing
                n146 = call "PH_PILS.enable extExp.vi"("i ref in"=w585, "Experiment.Experiment"=w581, "error in"=w584) -> ("i ref out"=w583:refnum<vi>, "error out"=w582:errorcluster)  [unwired: 15 in]
              }
              n147 = call "PH_PILS.set Doors ExtExp.vi"("i ref in"=w568, "error in"=w567) -> ("i ref out"=w566:refnum<vi>, "error out"=w565:errorcluster)  [unwired: 16 in]
              n148 = call "PH_PILS.vis extExpKnob.vi"("i ref in"=w566, "error IO"=w565) -> ("i ref out"=w562:refnum<vi>, "error out"=w564:errorcluster)  [unwired: 16 in]
              n149 = call "PH_PILS.vis MainAmpEnablingKnob.vi"("i ref in"=w562, "error IO"=w564) -> ("i ref out"=w561:refnum<vi>, "error out"=w563:errorcluster)  [unwired: 16 in]
            }
            frame Error {
            }
          }
          n150 = call "BaseProcess.set event status.vi"("i ref in"=w548, "EventStatus"=w557, "error in (no error)"=w549) -> ("i ref out"=w555:refnum<vi>, "error out"=w554:errorcluster)  [unwired: 14 in, 1 out]
          n151 = case shown="No Error" w554 {
            selector: w554 -> [_ w590]
            tunnel: [_ w588] -> w559
            frame No Error {
            }
            frame Error {
              n152 = Unbundle By Name(w590) -> ("source"=w589:string)
              n153 = call-poly "CoreLib.data 2 byte array.vi"("string"=w589) -> ("byteArray out"=w588:T1)  [unwired: 18 in]
            }
          }
          n154 = Unbundle By Name(w554) -> ("code"=w558:i32)
          n155 = Bundle By Name(cluster=w553, "Data"=w559, "Error #"=w558) -> (w552:T2)
        }
        frame "_Boolean" {
          n156 = call "CAEObj.unfold trend data.vi"("i ref in"=w600, "raw trend data"=w605) -> ("quality"=w593:i32, "no link"=w595:bool, "data"=w594:i8[], "serviceName"=w591:string, "typeDescriptor"=w592:string, "error out"=w596:errorcluster)  [unwired: 9 in, 3 out]
          n157 = case shown="No Error" w596 {
            tunnel: w599 -> [w620 w621]
            tunnel: [w611 w622] -> w597
            tunnel: [w609 w621] -> w598
            tunnel: w600 -> [w619 w622]
            tunnel: w595 -> [w616 _]
            tunnel: w592 -> [w615 _]
            tunnel: w594 -> [w618 _]
            tunnel: w593 -> [w617 _]
            tunnel: w591 -> [w614 _]
            frame No Error {
              n158 = call "PH_DIM.get Boolean.vi"("no link"=w616, "typeDescriptor"=w615, "data"=w618, "quality"=w617) -> ("Value"=w613:i32)
              n159 = call "PH_PILS.PC _Boolean.vi"("i ref in"=w619, "serviceName"=w614, "Value"=w613, "error IO"=w620) -> ("i ref out"=w612:refnum<vi>, "error out"=w610:errorcluster)  [unwired: 14 in]
              n160 = call "PH_PILS.ExtShutters.vi"("i ref in"=w612, "error IO"=w610) -> ("i ref out"=w611:refnum<vi>, "error out"=w609:errorcluster)  [unwired: 16 in]
            }
            frame Error {
            }
          }
          n161 = call "BaseProcess.set event status.vi"("i ref in"=w597, "EventStatus"=w606, "error in (no error)"=w598) -> ("i ref out"=w604:refnum<vi>, "error out"=w603:errorcluster)  [unwired: 14 in, 1 out]
          n162 = Unbundle By Name(w603) -> ("code"=w607:i32)
          n163 = case shown="Error" w603 {
            selector: w603 -> [_ w625]
            tunnel: [_ w623] -> w608
            frame No Error {
            }
            frame Error {
              n164 = Unbundle By Name(w625) -> ("source"=w624:string)
              n165 = call-poly "CoreLib.data 2 byte array.vi"("string"=w624) -> ("byteArray out"=w623:T1)  [unwired: 18 in]
            }
          }
          n166 = Bundle By Name(cluster=w602, "Data"=w608, "Error #"=w607) -> (w601:T2)
        }
        frame "_SpecialBoolean" {
          n167 = call "CAEObj.unfold trend data.vi"("i ref in"=w635, "raw trend data"=w640) -> ("quality"=w628:i32, "no link"=w630:bool, "data"=w629:i8[], "serviceName"=w626:string, "typeDescriptor"=w627:string, "error out"=w631:errorcluster)  [unwired: 9 in, 3 out]
          n168 = case shown="No Error" w631 {
            tunnel: w634 -> [w655 w656]
            tunnel: [w646 w657] -> w632
            tunnel: [w644 w656] -> w633
            tunnel: w635 -> [w654 w657]
            tunnel: w630 -> [w651 _]
            tunnel: w627 -> [w650 _]
            tunnel: w629 -> [w653 _]
            tunnel: w628 -> [w652 _]
            tunnel: w626 -> [w649 _]
            frame No Error {
              n169 = call "PH_DIM.get Boolean.vi"("no link"=w651, "typeDescriptor"=w650, "data"=w653, "quality"=w652) -> ("Value"=w648:i32)
              n170 = call "PH_PILS.PC _SpecialBoolean.vi"("i ref in"=w654, "serviceName"=w649, "Value"=w648, "error IO"=w655) -> ("i ref out"=w647:refnum<vi>, "error out"=w645:errorcluster)  [unwired: 14 in]
              n171 = call "PH_PILS.vis LaserEnablingKnob.vi"("i ref in"=w647, "error IO"=w645) -> ("i ref out"=w646:refnum<vi>, "error out"=w644:errorcluster)  [unwired: 16 in]
            }
            frame Error {
            }
          }
          n172 = call "BaseProcess.set event status.vi"("i ref in"=w632, "EventStatus"=w641, "error in (no error)"=w633) -> ("i ref out"=w639:refnum<vi>, "error out"=w638:errorcluster)  [unwired: 14 in, 1 out]
          n173 = Unbundle By Name(w638) -> ("code"=w642:i32)
          n174 = case shown="Error" w638 {
            selector: w638 -> [_ w660]
            tunnel: [_ w658] -> w643
            frame No Error {
            }
            frame Error {
              n175 = Unbundle By Name(w660) -> ("source"=w659:string)
              n176 = call-poly "CoreLib.data 2 byte array.vi"("string"=w659) -> ("byteArray out"=w658:T1)  [unwired: 18 in]
            }
          }
          n177 = Bundle By Name(cluster=w637, "Data"=w643, "Error #"=w642) -> (w636:T2)
        }
        frame "_Tristate2Run" {
          n178 = call "CAEObj.unfold trend data.vi"("i ref in"=w670, "raw trend data"=w675) -> ("quality"=w663:i32, "no link"=w665:bool, "data"=w664:i8[], "serviceName"=w661:string, "typeDescriptor"=w662:string, "error out"=w666:errorcluster)  [unwired: 9 in, 3 out]
          n179 = case shown="No Error" w666 {
            tunnel: w669 -> [w684 w712]
            tunnel: [w683 w713] -> w667
            tunnel: [w682 w712] -> w668
            tunnel: w670 -> [w685 w713]
            tunnel: w665 -> [w694 _]
            tunnel: w662 -> [w693 _]
            tunnel: w664 -> [w696 _]
            tunnel: w663 -> [w695 _]
            tunnel: w661 -> [w681 _]
            frame No Error {
              n180 = call "PH_PILS.get i attribute.vi"("i ref in"=w685, "error in (no error)"=w684) -> ("i ref out"=w686:refnum<vi>, "i attribute"=w688:T8, "error out"=w687:errorcluster)  [unwired: 15 in]
              n181 = call "PH_DIM.get Boolean.vi"("no link"=w694, "typeDescriptor"=w693, "data"=w696, "quality"=w695) -> ("Value"=w680:i32)
              n182 = case shown="1" w680 {
                selector: w680 -> [w697 _]
                tunnel: [w697 3 ("Value")] -> w679
                frame 0, Default {
                }
                frame 1 {
                }
              }
              n183 = Unbundle By Name(w688) -> ("Tristate2Run GUI Refs"=w692:refnum<vi>[])
              n184 = for {
                tunnel: w692 -> [w708] mode=indexing
                shift-right: [w711] -> w689
                shift-left: w687 -> [w710]
                tunnel: [w709] -> w690 mode=indexing
                n185 = property class="ColBox"(reference=w708, error in=w710) -> (error out=w711:errorcluster, "Label.Text"=w709:string)  [unwired: 1 out]
              }
              n186 = Search 1D Array(1D array=w690, element=w681) -> (index of element=w691:i32)  [unwired: 1 in]
              n187 = case shown="Default" w691 {
                selector: w691 -> [_ w705]
                tunnel: w686 -> [w700 w704]
                tunnel: [w700 w704] -> w683
                tunnel: [w699 w703] -> w682
                tunnel: w689 -> [w699 w706]
                tunnel: w692 -> [_ w707]
                tunnel: w679 -> [_ w701]
                frame -1 {
                }
                frame Default {
                  n188 = Index Array(array=w707, index=w705) -> (element=w702:refnum<vi>)
                  n189 = call "PH_GUI.set color GUI object.vi"("GUI object Ref"=w702, "State"=w701, "error in (no error)"=w706) -> ("error out"=w703:errorcluster)  [unwired: 16 in]
                }
              }
            }
            frame Error {
            }
          }
          n190 = call "BaseProcess.set event status.vi"("i ref in"=w667, "EventStatus"=w676, "error in (no error)"=w668) -> ("i ref out"=w674:refnum<vi>, "error out"=w673:errorcluster)  [unwired: 14 in, 1 out]
          n191 = Unbundle By Name(w673) -> ("code"=w677:i32)
          n192 = case shown="Error" w673 {
            selector: w673 -> [_ w716]
            tunnel: [_ w714] -> w678
            frame No Error {
            }
            frame Error {
              n193 = Unbundle By Name(w716) -> ("source"=w715:string)
              n194 = call-poly "CoreLib.data 2 byte array.vi"("string"=w715) -> ("byteArray out"=w714:T1)  [unwired: 18 in]
            }
          }
          n195 = Bundle By Name(cluster=w672, "Data"=w678, "Error #"=w677) -> (w671:T2)
        }
        frame "_TristateNormal" {
          n196 = call "CAEObj.unfold trend data.vi"("i ref in"=w726, "raw trend data"=w731) -> ("quality"=w719:i32, "no link"=w721:bool, "data"=w720:i8[], "serviceName"=w717:string, "typeDescriptor"=w718:string, "error out"=w722:errorcluster)  [unwired: 9 in, 3 out]
          n197 = case shown="No Error" w722 {
            tunnel: w725 -> [w752 w759]
            tunnel: [w741 w760] -> w723
            tunnel: [w743 w759] -> w724
            tunnel: w726 -> [w751 w760]
            tunnel: w721 -> [w756 _]
            tunnel: w718 -> [w755 _]
            tunnel: w720 -> [w758 _]
            tunnel: w719 -> [w757 _]
            tunnel: w717 -> [w750 _]
            frame No Error {
              n198 = call "PH_DIM.get Boolean.vi"("no link"=w756, "typeDescriptor"=w755, "data"=w758, "quality"=w757) -> ("Value"=w749:i32)
              n199 = call "PH_PILS.PC _TristateNormal.vi"("i ref in"=w751, "serviceName"=w750, "Value"=w749, "error IO"=w752) -> ("i ref out"=w754:refnum<vi>, "error out"=w753:errorcluster)  [unwired: 14 in]
              n200 = call "PH_PILS.set HV Warnlamp.vi"("i ref in"=w754, "error in (no error)"=w753) -> ("i ref out"=w748:refnum<vi>, "error out"=w747:errorcluster)  [unwired: 16 in]
              n201 = call "PH_PILS.enable PreAmp.vi"("i ref in"=w748, "error in"=w747) -> ("i ref out"=w736:refnum<vi>, "error out"=w739:errorcluster)  [unwired: 16 in]
              n202 = call "PH_PILS.set Radiation Shutters.vi"("i ref in"=w736, "error in"=w739) -> ("i ref out"=w737:refnum<vi>, "error out"=w740:errorcluster)  [unwired: 16 in]
              n203 = call "PH_PILS.enable MainAmp.vi"("i ref in"=w737, "error in"=w740) -> ("i ref out"=w735:refnum<vi>, "error out"=w738:errorcluster)  [unwired: 16 in]
              n204 = call "PH_PILS.vis HVroomLockKnob.vi"("i ref in"=w735, "error IO"=w738) -> ("i ref out"=w746:refnum<vi>, "error out"=w745:errorcluster)  [unwired: 16 in]
              n205 = call "PH_PILS.vis PreAmpEnablingKnob.vi"("i ref in"=w746, "error IO"=w745) -> ("i ref out"=w742:refnum<vi>, "error out"=w744:errorcluster)  [unwired: 16 in]
              n206 = call "PH_PILS.vis MainAmpEnablingKnob.vi"("i ref in"=w742, "error IO"=w744) -> ("i ref out"=w741:refnum<vi>, "error out"=w743:errorcluster)  [unwired: 16 in]
            }
            frame Error {
            }
          }
          n207 = call "BaseProcess.set event status.vi"("i ref in"=w723, "EventStatus"=w732, "error in (no error)"=w724) -> ("i ref out"=w730:refnum<vi>, "error out"=w729:errorcluster)  [unwired: 14 in, 1 out]
          n208 = Unbundle By Name(w729) -> ("code"=w733:i32)
          n209 = case shown="Error" w729 {
            selector: w729 -> [_ w763]
            tunnel: [_ w761] -> w734
            frame No Error {
            }
            frame Error {
              n210 = Unbundle By Name(w763) -> ("source"=w762:string)
              n211 = call-poly "CoreLib.data 2 byte array.vi"("string"=w762) -> ("byteArray out"=w761:T1)  [unwired: 18 in]
            }
          }
          n212 = Bundle By Name(cluster=w728, "Data"=w734, "Error #"=w733) -> (w727:T2)
        }
        frame "_PP" {
          n213 = call "CAEObj.unfold trend data.vi"("i ref in"=w773, "raw trend data"=w778) -> ("quality"=w766:i32, "no link"=w768:bool, "data"=w767:i8[], "serviceName"=w764:string, "typeDescriptor"=w765:string, "error out"=w769:errorcluster)  [unwired: 9 in, 3 out]
          n214 = case shown="No Error" w769 {
            tunnel: w772 -> [w793 w798]
            tunnel: [w784 w799] -> w770
            tunnel: [w782 w798] -> w771
            tunnel: w773 -> [w792 w799]
            tunnel: w768 -> [w795 _]
            tunnel: w765 -> [w794 _]
            tunnel: w767 -> [w797 _]
            tunnel: w766 -> [w796 _]
            tunnel: w764 -> [w786 _]
            frame No Error {
              n215 = call "PH_DIM.get Boolean.vi"("no link"=w795, "typeDescriptor"=w794, "data"=w797, "quality"=w796) -> ("Value"=w791:i32)
              n216 = call "PH_PILS.PC _PSUs.vi"("i ref in"=w792, "serviceName"=w786, "Value"=w791, "error IO"=w793) -> ("i ref out"=w789:refnum<vi>, "error out"=w790:errorcluster)  [unwired: 14 in]
              n217 = call "PH_PILS.set PPMA.vi"("i ref in"=w789, "Tagname"=w786, "error in"=w790) -> ("i ref out"=w788:refnum<vi>, "error out"=w787:errorcluster)  [unwired: 15 in]
              n218 = call "PH_PILS.set PPPA.vi"("i ref in"=w788, "Tagname"=w786, "error in"=w787) -> ("i ref out"=w785:refnum<vi>, "error out"=w783:errorcluster)  [unwired: 15 in]
              n219 = call "PH_PILS.set HV Greenlamp.vi"("i ref in"=w785, "error in (no error)"=w783) -> ("i ref out"=w784:refnum<vi>, "error out"=w782:errorcluster)  [unwired: 16 in]
            }
            frame Error {
            }
          }
          n220 = call "BaseProcess.set event status.vi"("i ref in"=w770, "EventStatus"=w779, "error in (no error)"=w771) -> ("i ref out"=w777:refnum<vi>, "error out"=w776:errorcluster)  [unwired: 14 in, 1 out]
          n221 = Unbundle By Name(w776) -> ("code"=w780:i32)
          n222 = case shown="Error" w776 {
            selector: w776 -> [_ w802]
            tunnel: [_ w800] -> w781
            frame No Error {
            }
            frame Error {
              n223 = Unbundle By Name(w802) -> ("source"=w801:string)
              n224 = call-poly "CoreLib.data 2 byte array.vi"("string"=w801) -> ("byteArray out"=w800:T1)  [unwired: 18 in]
            }
          }
          n225 = Bundle By Name(cluster=w775, "Data"=w781, "Error #"=w780) -> (w774:T2)
        }
        frame "_Tristate_EO_Like" {
          n226 = call "CAEObj.unfold trend data.vi"("i ref in"=w812, "raw trend data"=w817) -> ("quality"=w805:i32, "no link"=w807:bool, "data"=w806:i8[], "serviceName"=w803:string, "typeDescriptor"=w804:string, "error out"=w808:errorcluster)  [unwired: 9 in, 3 out]
          n227 = case shown="No Error" w808 {
            tunnel: w811 -> [w826 w831]
            tunnel: [w822 w832] -> w809
            tunnel: [w821 w831] -> w810
            tunnel: w812 -> [w825 w832]
            tunnel: w807 -> [w828 _]
            tunnel: w804 -> [w827 _]
            tunnel: w806 -> [w830 _]
            tunnel: w805 -> [w829 _]
            tunnel: w803 -> [w824 _]
            frame No Error {
              n228 = call "PH_DIM.get Boolean.vi"("no link"=w828, "typeDescriptor"=w827, "data"=w830, "quality"=w829) -> ("Value"=w823:i32)
              n229 = call "PH_PILS.PC _TristateEOLike.vi"("i ref in"=w825, "serviceName"=w824, "Value"=w823, "error IO"=w826) -> ("i ref out"=w822:refnum<vi>, "error out"=w821:errorcluster)  [unwired: 14 in]
            }
            frame Error {
            }
          }
          n230 = call "BaseProcess.set event status.vi"("i ref in"=w809, "EventStatus"=w818, "error in (no error)"=w810) -> ("i ref out"=w816:refnum<vi>, "error out"=w815:errorcluster)  [unwired: 14 in, 1 out]
          n231 = Unbundle By Name(w815) -> ("code"=w819:i32)
          n232 = case shown="Error" w815 {
            selector: w815 -> [_ w835]
            tunnel: [_ w833] -> w820
            frame No Error {
            }
            frame Error {
              n233 = Unbundle By Name(w835) -> ("source"=w834:string)
              n234 = call-poly "CoreLib.data 2 byte array.vi"("string"=w834) -> ("byteArray out"=w833:T1)  [unwired: 18 in]
            }
          }
          n235 = Bundle By Name(cluster=w814, "Data"=w820, "Error #"=w819) -> (w813:T2)
        }
        frame "_DoorTags" {
          n236 = call "CAEObj.unfold trend data.vi"("i ref in"=w845, "raw trend data"=w850) -> ("quality"=w838:i32, "no link"=w840:bool, "data"=w839:i8[], "serviceName"=w836:string, "typeDescriptor"=w837:string, "error out"=w841:errorcluster)  [unwired: 9 in, 3 out]
          n237 = case shown="No Error" w841 {
            tunnel: w844 -> [w889 w894]
            tunnel: [w858 w895] -> w842
            tunnel: [w860 w894] -> w843
            tunnel: w845 -> [w888 w895]
            tunnel: w840 -> [w891 _]
            tunnel: w837 -> [w890 _]
            tunnel: w839 -> [w893 _]
            tunnel: w838 -> [w892 _]
            tunnel: w836 -> [w864 _]
            frame No Error {
              n238 = call "PH_DIM.get Boolean.vi"("no link"=w891, "typeDescriptor"=w890, "data"=w893, "quality"=w892) -> ("Value"=w887:i32)
              n239 = call "PH_PILS.PC _DoorTags.vi"("i ref in"=w888, "serviceName"=w864, "Value"=w887, "error IO"=w889) -> ("i ref out"=w884:refnum<vi>, "error out"=w886:errorcluster)  [unwired: 14 in]
              n240 = call "PH_PILS.enable Laser.vi"("i ref in"=w884, "error in"=w886) -> ("i ref out"=w883:refnum<vi>, "error out"=w885:errorcluster)  [unwired: 16 in]
              n241 = call "PH_PILS.Action _Cerpass.vi"("i ref in"=w883, "Service Name"=w864, "error in"=w885) -> ("i ref out"=w882:refnum<vi>, "error out"=w881:errorcluster)  [unwired: 15 in]
              n242 = call "PH_PILS.set Doors Laserbay.vi"("i ref in"=w882, "Service Name"=w864, "error in"=w881) -> ("i ref out"=w880:refnum<vi>, "error out"=w879:errorcluster)  [unwired: 15 in]
              n243 = call "PH_PILS.set Doors Laserlab.vi"("i ref in"=w880, "String"=w864, "error in"=w879) -> ("i ref out"=w878:refnum<vi>, "error out"=w877:errorcluster)  [unwired: 15 in]
              n244 = call "PH_PILS.set Doors Beam Diag.vi"("i ref in"=w878, "Service Name"=w864, "error in"=w877) -> ("i ref out"=w876:refnum<vi>, "error out"=w875:errorcluster)  [unwired: 15 in]
              n245 = call "PH_PILS.set Doors HV room.vi"("i ref in"=w876, "Service Name"=w864, "error in"=w875) -> ("i ref out"=w874:refnum<vi>, "error out"=w873:errorcluster)  [unwired: 15 in]
              n246 = call "PH_PILS.set Doors ELT room.vi"("i ref in"=w874, "Service Name"=w864, "error in"=w873) -> ("i ref out"=w872:refnum<vi>, "error out"=w871:errorcluster)  [unwired: 15 in]
              n247 = call "PH_PILS.enable PreAmp.vi"("i ref in"=w872, "error in"=w871) -> ("i ref out"=w857:refnum<vi>, "error out"=w855:errorcluster)  [unwired: 16 in]
              n248 = call "PH_PILS.set Radiation Shutters.vi"("i ref in"=w857, "error in"=w855) -> ("i ref out"=w856:refnum<vi>, "error out"=w854:errorcluster)  [unwired: 16 in]
              n249 = call "PH_PILS.enable MainAmp.vi"("i ref in"=w856, "error in"=w854) -> ("i ref out"=w870:refnum<vi>, "error out"=w869:errorcluster)  [unwired: 16 in]
              n250 = call "PH_PILS.set Doors ExtExp.vi"("i ref in"=w870, "error in"=w869) -> ("i ref out"=w868:refnum<vi>, "error out"=w867:errorcluster)  [unwired: 16 in]
              n251 = call "PH_PILS.set MAGroudSticks.vi"("i ref in"=w868, "error in"=w867) -> ("i ref out"=w866:refnum<vi>, "error out"=w865:errorcluster)  [unwired: 16 in]
              n252 = call "PH_PILS.vis LaserEnablingKnob.vi"("i ref in"=w866, "error IO"=w865) -> ("i ref out"=w863:refnum<vi>, "error out"=w862:errorcluster)  [unwired: 16 in]
              n253 = call "PH_PILS.vis PreAmpEnablingKnob.vi"("i ref in"=w863, "error IO"=w862) -> ("i ref out"=w859:refnum<vi>, "error out"=w861:errorcluster)  [unwired: 16 in]
              n254 = call "PH_PILS.vis MainAmpEnablingKnob.vi"("i ref in"=w859, "error IO"=w861) -> ("i ref out"=w858:refnum<vi>, "error out"=w860:errorcluster)  [unwired: 16 in]
            }
            frame Error {
            }
          }
          n255 = call "BaseProcess.set event status.vi"("i ref in"=w842, "EventStatus"=w851, "error in (no error)"=w843) -> ("i ref out"=w849:refnum<vi>, "error out"=w848:errorcluster)  [unwired: 14 in, 1 out]
          n256 = Unbundle By Name(w848) -> ("code"=w852:i32)
          n257 = case shown="Error" w848 {
            selector: w848 -> [_ w898]
            tunnel: [_ w896] -> w853
            frame No Error {
            }
            frame Error {
              n258 = Unbundle By Name(w898) -> ("source"=w897:string)
              n259 = call-poly "CoreLib.data 2 byte array.vi"("string"=w897) -> ("byteArray out"=w896:T1)  [unwired: 18 in]
            }
          }
          n260 = Bundle By Name(cluster=w847, "Data"=w853, "Error #"=w852) -> (w846:T2)
        }
        frame "_ShutterTags" {
          n261 = call "CAEObj.unfold trend data.vi"("i ref in"=w908, "raw trend data"=w913) -> ("quality"=w901:i32, "no link"=w903:bool, "data"=w902:i8[], "serviceName"=w899:string, "typeDescriptor"=w900:string, "error out"=w904:errorcluster)  [unwired: 9 in, 3 out]
          n262 = case shown="No Error" w904 {
            tunnel: w907 -> [w930 w935]
            tunnel: [w924 w936] -> w905
            tunnel: [w923 w935] -> w906
            tunnel: w908 -> [w929 w936]
            tunnel: w903 -> [w932 _]
            tunnel: w900 -> [w931 _]
            tunnel: w902 -> [w934 _]
            tunnel: w901 -> [w933 _]
            tunnel: w899 -> [w928 _]
            frame No Error {
              n263 = call "PH_DIM.get Boolean.vi"("no link"=w932, "typeDescriptor"=w931, "data"=w934, "quality"=w933) -> ("Value"=w927:i32)
              n264 = call "PH_PILS.PC _ShutterTags.vi"("i ref in"=w929, "serviceName"=w928, "Value"=w927, "error IO"=w930) -> ("i ref out"=w921:refnum<vi>, "error out"=w922:errorcluster)  [unwired: 14 in]
              n265 = call "PH_PILS.set Laser Shutters.vi"("i ref in"=w921, "error in"=w922) -> ("i ref out"=w926:refnum<vi>, "error out"=w925:errorcluster)  [unwired: 16 in]
              n266 = call "PH_PILS.enable PreAmp.vi"("i ref in"=w926, "error in"=w925) -> ("i ref out"=w920:refnum<vi>, "error out"=w918:errorcluster)  [unwired: 16 in]
              n267 = call "PH_PILS.set Radiation Shutters.vi"("i ref in"=w920, "error in"=w918) -> ("i ref out"=w919:refnum<vi>, "error out"=w917:errorcluster)  [unwired: 16 in]
              n268 = call "PH_PILS.vis PreAmpEnablingKnob.vi"("i ref in"=w919, "error IO"=w917) -> ("i ref out"=w924:refnum<vi>, "error out"=w923:errorcluster)  [unwired: 16 in]
            }
            frame Error {
            }
          }
          n269 = call "BaseProcess.set event status.vi"("i ref in"=w905, "EventStatus"=w914, "error in (no error)"=w906) -> ("i ref out"=w912:refnum<vi>, "error out"=w911:errorcluster)  [unwired: 14 in, 1 out]
          n270 = Unbundle By Name(w911) -> ("code"=w915:i32)
          n271 = case shown="Error" w911 {
            selector: w911 -> [_ w939]
            tunnel: [_ w937] -> w916
            frame No Error {
            }
            frame Error {
              n272 = Unbundle By Name(w939) -> ("source"=w938:string)
              n273 = call-poly "CoreLib.data 2 byte array.vi"("string"=w938) -> ("byteArray out"=w937:T1)  [unwired: 18 in]
            }
          }
          n274 = Bundle By Name(cluster=w910, "Data"=w916, "Error #"=w915) -> (w909:T2)
        }
        frame "_SwitchKnobs" {
          n275 = call "CAEObj.unfold trend data.vi"("i ref in"=w949, "raw trend data"=w954) -> ("quality"=w942:i32, "no link"=w944:bool, "data"=w943:i8[], "serviceName"=w940:string, "typeDescriptor"=w941:string, "error out"=w945:errorcluster)  [unwired: 9 in, 3 out]
          n276 = case shown="No Error" w945 {
            tunnel: w948 -> [w963 w968]
            tunnel: [w958 w969] -> w946
            tunnel: [w959 w968] -> w947
            tunnel: w949 -> [w962 w969]
            tunnel: w944 -> [w965 _]
            tunnel: w941 -> [w964 _]
            tunnel: w943 -> [w967 _]
            tunnel: w942 -> [w966 _]
            tunnel: w940 -> [w960 _]
            frame No Error {
              n277 = call "PH_DIM.get Boolean.vi"("no link"=w965, "typeDescriptor"=w964, "data"=w967, "quality"=w966) -> ("Value"=w961:i32)
              n278 = call "PH_PILS.PC _SwitchKnob.vi"("i ref in"=w962, "serviceName"=w960, "Value"=w961, "error IO"=w963) -> ("i ref out"=w958:refnum<vi>, "error out"=w959:errorcluster)  [unwired: 14 in]
            }
            frame Error {
            }
          }
          n279 = call "BaseProcess.set event status.vi"("i ref in"=w946, "EventStatus"=w955, "error in (no error)"=w947) -> ("i ref out"=w953:refnum<vi>, "error out"=w952:errorcluster)  [unwired: 14 in, 1 out]
          n280 = Unbundle By Name(w952) -> ("code"=w956:i32)
          n281 = case shown="Error" w952 {
            selector: w952 -> [_ w972]
            tunnel: [_ w970] -> w957
            frame No Error {
            }
            frame Error {
              n282 = Unbundle By Name(w972) -> ("source"=w971:string)
              n283 = call-poly "CoreLib.data 2 byte array.vi"("string"=w971) -> ("byteArray out"=w970:T1)  [unwired: 18 in]
            }
          }
          n284 = Bundle By Name(cluster=w951, "Data"=w957, "Error #"=w956) -> (w950:T2)
        }
        frame "_Mercury" {
          n285 = call "CAEObj.unfold trend data.vi"("i ref in"=w982, "raw trend data"=w987) -> ("quality"=w975:i32, "no link"=w977:bool, "data"=w976:i8[], "serviceName"=w973:string, "typeDescriptor"=w974:string, "error out"=w978:errorcluster)  [unwired: 9 in, 3 out]
          n286 = case shown="No Error" w978 {
            tunnel: w981 -> [w998 w1035]
            tunnel: [w996 w1036] -> w979
            tunnel: [w995 w1035] -> w980
            tunnel: w982 -> [w999 w1036]
            tunnel: w977 -> [w1004 _]
            tunnel: w974 -> [w1003 _]
            tunnel: w976 -> [w1006 _]
            tunnel: w975 -> [w1005 _]
            tunnel: w973 -> [w1001 _]
            frame No Error {
              n287 = call "PH_PILS.get i attribute.vi"("i ref in"=w999, "error in (no error)"=w998) -> ("i ref out"=w996:refnum<vi>, "i attribute"=w994:T8, "error out"=w997:errorcluster)  [unwired: 15 in]
              n288 = Unbundle By Name(w994) -> ("Mercury"=w993:refnum<vi>)
              n289 = call "PH_Beckhoff_PP_Control.get PP Mercury Tagname.vi"("PP Mercury Tag"=PH_Beckhoff_PP_Control.PP_Mercury_Tags."Status") -> ("PP Mercury Tagname"=w1000:string)
              n290 = Equal?(x=w1001, y=w1000) -> (x = y?=w991:bool)
              n291 = Not A Number/Path/Refnum?(number/path/refnum=w993) -> (NaN/Path/Refnum?=w992:bool)
              n292 = case shown="False" w992 {
                tunnel: w1006 -> [w1014 _]
                tunnel: w1005 -> [w1013 _]
                tunnel: w1004 -> [w1012 _]
                tunnel: w1003 -> [w1011 _]
                tunnel: w997 -> [w1010 w1034]
                tunnel: [w1009 w1034] -> w995
                tunnel: w993 -> [w1008 _]
                tunnel: w991 -> [w1007 _]
                frame False {
                  n293 = case shown="True" w1007 {
                    tunnel: w1014 -> [w1023 w1033]
                    tunnel: w1013 -> [w1022 _]
                    tunnel: w1012 -> [w1021 w1028]
                    tunnel: w1011 -> [w1020 w1032]
                    tunnel: w1010 -> [w1019 w1030]
                    tunnel: [w1018 w1029] -> w1009
                    tunnel: w1008 -> [w1017 w1031]
                    frame False {
                      n294 = call "PH_DIM.get String.vi"("no link"=w1021, "typeDescriptor"=w1020, "data"=w1023, "quality"=w1022) -> ("Output String"=w1016:string)
                      n295 = property class="ColBox"(reference=w1017, error in=w1019, "Caption.Text"=w1016, "Caption.Visible"=TRUE) -> (error out=w1018:errorcluster)  [unwired: 1 out]
                    }
                    frame True {
                      n296 = call "PH_StatusHandler.get Status DIM Service.vi"("no link"=w1028, "typeDescriptor"=w1032, "data"=w1033) -> ("Status"=w1027:T12)  [unwired: 1 in]
                      n297 = To Long Integer(number=w1027) -> (32bit integer=w1025:i32)
                      n298 = call "PH_GUI.Sevencolor.vi"("State"=w1025) -> ("Color Box"=w1026:u32)
                      n299 = property class="ColBox"(reference=w1031, error in=w1030, "Value"=w1026, "Blinking"=w1028, "Caption.Visible"=TRUE) -> (error out=w1029:errorcluster)  [unwired: 1 out]
                    }
                  }
                }
                frame True {
                }
              }
            }
            frame Error {
            }
          }
          n300 = call "BaseProcess.set event status.vi"("i ref in"=w979, "EventStatus"=w988, "error in (no error)"=w980) -> ("i ref out"=w986:refnum<vi>, "error out"=w985:errorcluster)  [unwired: 14 in, 1 out]
          n301 = Unbundle By Name(w985) -> ("code"=w989:i32)
          n302 = case shown="Error" w985 {
            selector: w985 -> [_ w1039]
            tunnel: [_ w1037] -> w990
            frame No Error {
            }
            frame Error {
              n303 = Unbundle By Name(w1039) -> ("source"=w1038:string)
              n304 = call-poly "CoreLib.data 2 byte array.vi"("string"=w1038) -> ("byteArray out"=w1037:T1)  [unwired: 18 in]
            }
          }
          n305 = Bundle By Name(cluster=w984, "Data"=w990, "Error #"=w989) -> (w983:T2)
        }
      }
    }
    frame Error {
    }
  }
  "answer cluster" <- w7
  "i ref out" <- w4
  "error out" <- w3
